vi "Write Value.vi"(8 "error in (no error)":errorcluster caption="entrée d'erreur (pas d'erreur)", 10 "Data":string, 11 "DAQmxTaskDOutput_Emulate en entrée":refnum<class "DAQmxTaskDOutput_Emulate.lvclass">) -> (0 "error out":errorcluster caption="sortie d'erreur", 3 "DAQmxTaskDOutput_Emulate en sortie":refnum<class "DAQmxTaskDOutput_Emulate.lvclass">)   [LabVIEW 2018, in "DAQmxTaskDOutput_Emulate.lvclass"]
uses:
  DAQmxTaskDOutput_Emulate.lvclass
  C:/Users/Sergey Denisov/Documents/REPS/TRANCON/Classes/DAQmxTasks/DAQmxTask.lvclass
  DAQmxTask.lvclass/DAQmxTask.ctl
  DAQmxTask.lvclass
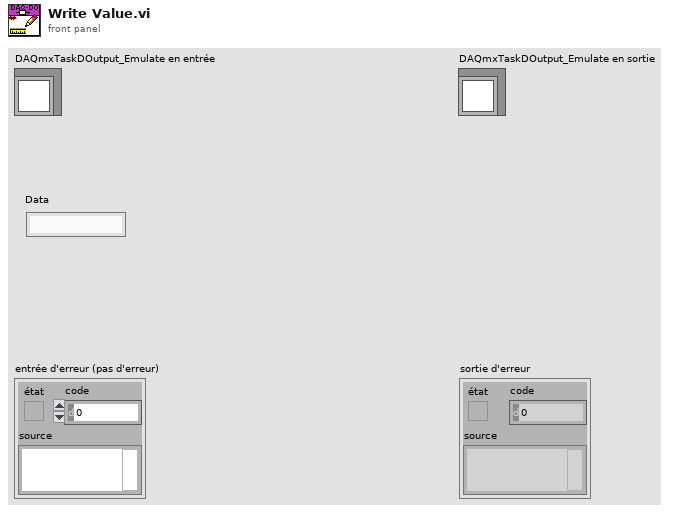
[diagram p1: front panel]
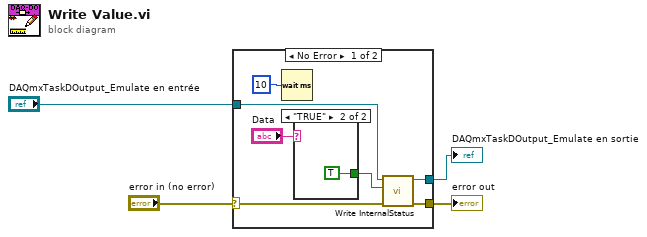
[diagram p0: block diagram]
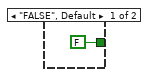
[diagram p2: hidden frame]
diagram:
  n1 = case shown="No Error" "error in (no error)" {
    selector: "error in (no error)" -> [w6 w15]
    tunnel: [w5 w15] -> w3
    tunnel: "DAQmxTaskDOutput_Emulate en entrée" -> [w9 w14]
    tunnel: [w8 w14] -> w1
    frame No Error {
      n2 = Wait (ms)(milliseconds to wait=u32 10) -> ()  [unwired: 1 out]
      n3 = case shown="\"TRUE\"" "Data" {
        tunnel: [FALSE TRUE] -> w7
        frame "FALSE", Default {
        }
        frame "TRUE" {
        }
      }
      n4 = call "Write InternalStatus.vi"("error in (no error)"=w6, "InternalStatus"=w7, "DAQmxTask in"=w9) -> ("error out"=w5:errorcluster, "DAQmxTask out"=w8:refnum<class "DAQmxTaskDOutput_Emulate.lvclass">)  [unwired: 7 in]
    }
    frame Error {
    }
  }
  "error out" <- w3
  "DAQmxTaskDOutput_Emulate en sortie" <- w1
